vi "UTF-8toGBK.vi"(10 "UTF-8":string="测试") -> (2 "GBK":string)   [LabVIEW 2017]
uses:
  kernel32.dll
panel:
  out "Unicode":string
  # "\"测试\"\nUTF-8   E6B5 8BE8 AF95\nUnicode 4B6D D58B \nGBK     B2E2 CAD4"
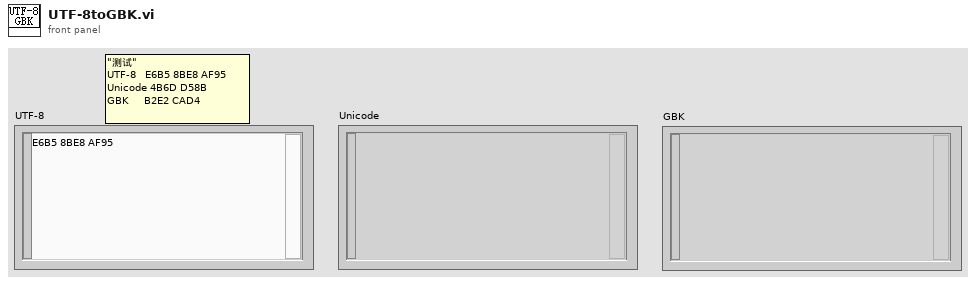
[diagram p1: front panel]
types:
  T1 = enum16{"big-endian, network order", "native, host order", "little-endian"}
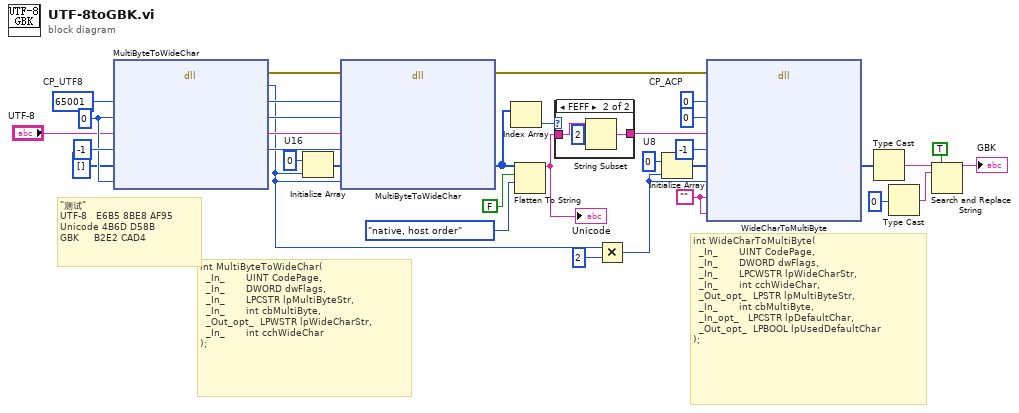
[diagram p0: block diagram]
diagram:
  w19 = u8 0  # U8
  w21 = u16 0  # U16
  w15 = u32 0  # CP_ACP
  w11 = ""
  w32 = 0 ("dwFlags")
  w31 = u32 65001  # CP_UTF8
  # "int MultiByteToWideChar(\n  _In_       UINT CodePage,\n  _In_       DWORD dwFlags,\n  _In_       LPCSTR lpMultiByteStr,\n  _In_       int cbMultiByte,\n  _Out_opt_  LPWSTR lpWideCharStr,\n  _In_       int cchWideChar\n);"
  # "int WideCharToMultiByte(\n  _In_       UINT CodePage,\n  _In_       DWORD dwFlags,\n  _In_       LPCWSTR lpWideCharStr,\n  _In_       int cchWideChar,\n  _Out_opt_  LPSTR lpMultiByteStr,\n  _In_       int cbMultiByte,\n  _In_opt_   LPCSTR lpDefaultChar,\n  _Out_opt_  LPBOOL lpUsedDefaultChar\n);"
  # "\"测试\"\nUTF-8   E6B5 8BE8 AF95\nUnicode 4B6D D58B \nGBK     B2E2 CAD4"
  n1 = dll-call lib="kernel32.dll" fn="MultiByteToWideChar"("CodePage"=w31, "dwFlags"=w32, "lpMultiByteStr"="UTF-8", "cbMultiByte"=-1, "lpWideCharStr"=u16[] [], "cchWideChar"=w32) -> (error out=w34:errorcluster, "返回类型"=w8:i32, "CodePage"=w28:u32, "dwFlags"=w29:i32, "lpMultiByteStr"=w30:string, "cbMultiByte"=w27:i32)  [unwired: 5 in, 1 out]
  n2 = Initialize Array(w21, w8) -> (w20:u16[])
  n3 = dll-call lib="kernel32.dll" fn="MultiByteToWideChar"(error in=w34, "CodePage"=w28, "dwFlags"=w29, "lpMultiByteStr"=w30, "cbMultiByte"=w27, "lpWideCharStr"=w20, "cchWideChar"=w8) -> (error out=w16:errorcluster, "lpWideCharStr"=w22:u16[])  [unwired: 8 in, 1 out]
  n4 = Index Array(array=w22) -> (element=w23:u16)  [unwired: 1 in]
  n5 = Flatten To String(anything=w22, prepend array or string size? (T)=FALSE ("预置数组或字符串大小？(T)"), byte order (0:big-endian, network order)=T1."native, host order" ("字节顺序(0:big-endian, network order)")) -> (data string=w10:string)  [unwired: 1 in, 2 out]
  "Unicode" <- w10
  n6 = case shown="FEFF" w23 {
    tunnel: w10 -> [w35 w37]
    tunnel: [w35 w36] -> w13
    frame Default {
    }
    frame 65279 {
      n7 = String Subset(string=w37, offset (0)=2 ("偏移量(0)")) -> (substring=w36:string)  [unwired: 1 in]
    }
  }
  n8 = Multiply(x=w8, y=2) -> (x*y=w7:i32)
  n9 = Initialize Array(w19, w7) -> (w18:u8[])
  n10 = dll-call lib="kernel32.dll" fn="WideCharToMultiByte"(error in=w16, "CodePage"=w15, "dwFlags"=0, "lpWideCharStr"=w13, "cchWideChar"=-1, "lpMultiByteStr"=w18, "cchMultiByte"=w7, "lpDefaultChar"=w11, "pfUsedDefaultChar"=w11) -> ("lpMultiByteStr"=w6:u8[])  [unwired: 10 in, 2 out]
  n11 = Type Cast(x=w6) -> (*(type *) &x=w3:string)  [unwired: 1 in]
  n12 = Type Cast(x=u8 0 ("元素")) -> (*(type *) &x=w5:string)  [unwired: 1 in]
  n13 = Search and Replace String(replace all?=TRUE ("替换全部？(F)"), input string=w3, search string=w5) -> (result string=→"GBK":string)  [unwired: 5 in, 3 out]
